vi "Mode_select_LED.vi"() -> (2 "Control_State":T1)   [LabVIEW 2020]
uses:
  LED_Control_States.ctl
  <vilib>/Rock Robotics/WPI/DriverStation/WPI_DriverStationRobotMode2.ctl
  Robot Global Data.vi
  Globals/Climber_Globals.vi
  Globals/Flywheel_Globals.vi
  Globals/Turret_Globals.vi
  Globals/Cowl_Globals.vi
  Globals/Sensor_Values.vi
  Globals/Autonomous_Globals.vi
  LED GLOBALS!!!.vi
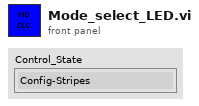
[diagram p1: front panel]
types:
  T1 = typedef "LED_Control_States.ctl" = enum16{"Config-Stripes", "swapperlines", "Rand", "Solid", "Flash-S", "Gradyent", "Move-Stripes", "Org-Rand", "Move-Point-Tail", "Flames", "Fade", "Alt-Colors"}
  T2 = typedef "WPI_DriverStationRobotMode2.ctl" = enum16{"Autonomous Disabled", "Autonomous Enabled", "Teleop Disabled", "Teleop Enabled", "Disconnected", "Finish", "Test Disabled", "Test Enabled", "Emergency Stopped"}
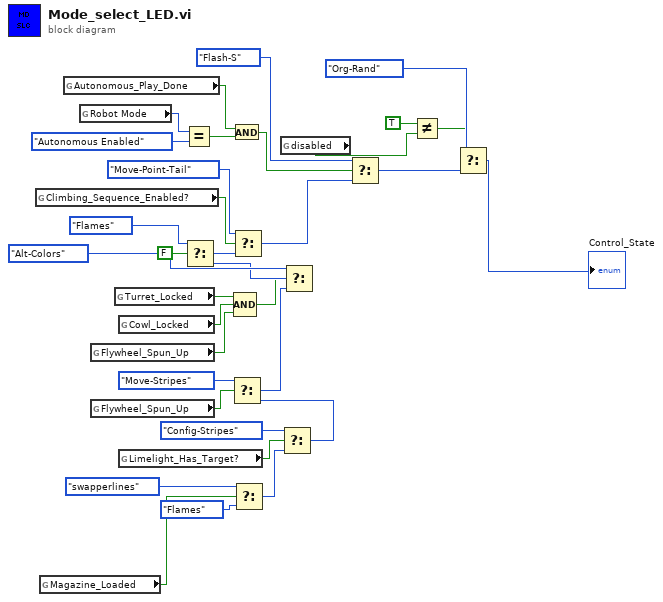
[diagram p0: block diagram]
diagram:
  n1 = global read "Climber_Globals.vi" "Climbing_Sequence_Enabled?"() -> (w20:bool)
  n2 = global read "Sensor_Values.vi" "Magazine_Loaded"() -> (w13:bool)
  n3 = global read "Autonomous_Globals.vi" "Autonomous_Play_Done"() -> (w11:bool)
  n4 = global read "Robot Global Data.vi" "Robot Mode"() -> (w22:T2)
  n5 = global read "Flywheel_Globals.vi" "Flywheel_Spun_Up"() -> (w7:bool)
  n6 = global read "Flywheel_Globals.vi" "Flywheel_Spun_Up"() -> (w17:bool)
  n7 = global read "Turret_Globals.vi" "Turret_Locked"() -> (w9:bool)
  n8 = global read "Cowl_Globals.vi" "Cowl_Locked"() -> (w8:bool)
  n9 = global read "Sensor_Values.vi" "Limelight_Has_Target?"() -> (w14:bool)
  n10 = Equal?(x=w22, y=WPI_DriverStationRobotMode2."Autonomous Enabled") -> (x = y?=w12:bool)
  n11 = And(x=w11, y=w12) -> (x .and. y?=w10:bool)
  n12 = Compound Arithmetic op=AND(w9, w8, w7) -> (w18:bool)
  n13 = Select(t=LED_Control_States."swapperlines" ("Control_State"), s=w13, f=LED_Control_States."Flames" ("Control_State")) -> (s? t:f=w16:T1)
  n14 = global read "LED GLOBALS!!!.vi" "disabled"() -> (w3:bool)
  n15 = Select(t=LED_Control_States."Config-Stripes" ("Control_State"), s=w14, f=w16) -> (s? t:f=w15:T1)
  n16 = Select(t=LED_Control_States."Move-Stripes" ("Control_State"), s=w17, f=w15) -> (s? t:f=w23:T1)
  n17 = Select(t=LED_Control_States."Alt-Colors" ("Control_State"), s=w18, f=w23) -> (s? t:f=w26:T1)
  n18 = Select(t=LED_Control_States."Flames" ("Control_State"), s=FALSE, f=w26) -> (s? t:f=w25:T1)
  n19 = Select(t=LED_Control_States."Move-Point-Tail" ("Control_State"), s=w20, f=w25) -> (s? t:f=w24:T1)
  n20 = Select(t=LED_Control_States."Flash-S" ("Control_State"), s=w10, f=w24) -> (s? t:f=w6:T1)
  n21 = Not Equal?(x=TRUE, y=w3) -> (x != y?=w2:bool)
  n22 = Select(t=LED_Control_States."Org-Rand" ("Control_State"), s=w2, f=w6) -> (s? t:f=→"Control_State":T1)
